vi "NI-DP_ListDevices.vi"() -> ()   [LabVIEW 2014, in "hse-network.lvlib"]
doc: "____\nHAMPEL SOFTWARE ENGINEERING v0.7.0 (2018-07-16 18:12)"
uses:
  hse-network.lvlib
panel:
  out "net address":u32
  out "name":string
  out "Devices":string[](array[string])
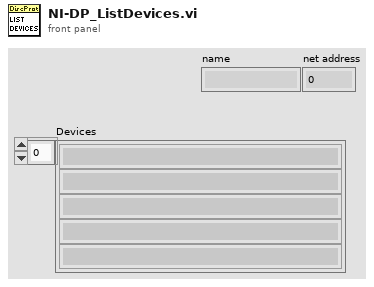
[diagram p1: front panel]
types:
  T1 = typedef "hse-network.lvlib/NI-DP__MessageStructure.ctl" = cluster{"Start of Message":string, "Command":T2, "Checksum(?) for P3,P4":string, "Always 0x02":string, "Model Code":string, "??? 1":string, "Serial":string, "Device Mac Address":string, "??? 2":string, "Param 1":string, "Param 2":string, "Param 3":string, "Param 4":string, "Checksum(?) for Network":string, "Device IP Address":string, "Device Subnet Mask":string, "Device DNS-Server":string, "Device Default Gateway":string, "??? 3":string, "End of Message":string}
  T2 = typedef "hse-network.lvlib/NI-DP__Commands.ctl" = u8
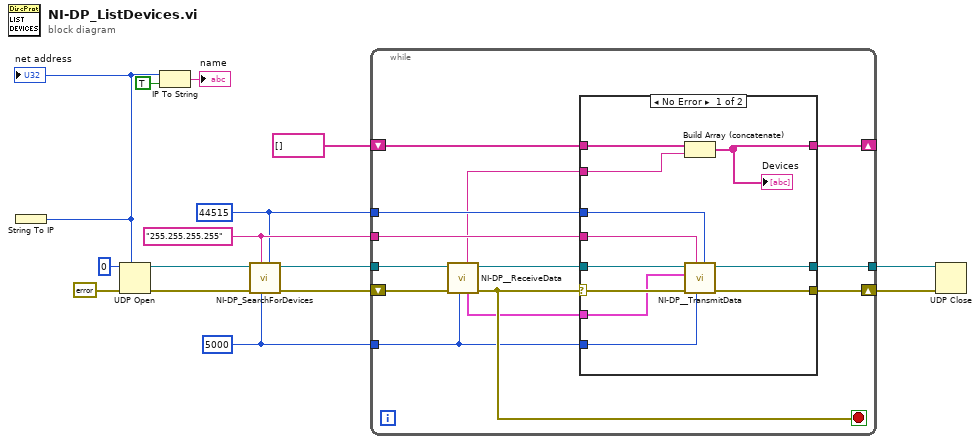
[diagram p0: block diagram]
diagram:
  w6 = u32 5000 ("timeout [ms]")
  w7 = u16 44515 ("RX Port No.")
  w8 = "255.255.255.255" ("IP to write to")
  n1 = String To IP() -> (0:w1:u32)  [unwired: 1 in]
  "net address" <- w1
  n2 = UDP Open(7:w1, 8:errorcluster {"status"=FALSE, "code"=0, "source"=""} ("error in (no error)"), 11:u16 0 ("port")) -> (port=w13:refnum<k16>, 0:w15:errorcluster)  [unwired: 2 in, 1 out]
  n3 = IP To String(1:TRUE ("dot notation? (F)"), 2:w1) -> (0:→"name":string)
  n4 = call "NI-DP_SearchForDevices.vi"("RX Port No."=w7, "timeout [ms]"=w6, "IP to write to"=w8, "error in (no error)"=w15, "UDP Network Connection in"=w13) -> ("error out"=w12:errorcluster, "UDP Network Connection out"=w11:refnum<k16>)  [unwired: 5 in]
  n5 = while {
    shift-right: [w26] -> w10
    shift-left: w12 -> [w28]
    tunnel: w11 -> [w25]
    tunnel: [w23] -> w9
    tunnel: w8 -> [w21]
    tunnel: w7 -> [w20]
    tunnel: w6 -> [w19]
    shift-right: [w18] -> _
    shift-left: string[] [] ("Array") -> [w17]
    stop <- w27 stop-if-true
    n6 = call "NI-DP__ReceiveData.vi"("timeout [ms]"=w19, "error in"=w28, "UDP Network Connection in"=w25) -> ("error out"=w27:errorcluster, "UDP Network Connection out"=w24:refnum<k16>, "UDP-NI Message"=w22:T1, "IP (MAC)"=w16:string)  [unwired: 3 in, 2 out]
    n7 = case shown="No Error" w27 {
      selector: w27 -> [w39 w41]
      tunnel: [w38 w41] -> w26
      tunnel: w24 -> [w37 w42]
      tunnel: [w36 w42] -> w23
      tunnel: w22 -> [w35 _]
      tunnel: w21 -> [w34 _]
      tunnel: w20 -> [w33 _]
      tunnel: w19 -> [w32 _]
      tunnel: [w29 w40] -> w18
      tunnel: w17 -> [w31 w40]
      tunnel: w16 -> [w30 _]
      frame No Error {
        n8 = Build Array (concatenate)(w31, w30) -> (w29:string[])
        "Devices" <- w29
        n9 = call "NI-DP__TransmitData.vi"("Port to write to"=w33, "timeout ms"=w32, "IP to write to"=w34, "error in"=w39, "UDP-NI__Message"=w35, "UDP Network Connection in"=w37) -> ("error out"=w38:errorcluster, "UDP Network Connection out"=w36:refnum<k16>)  [unwired: 4 in]
      }
      frame Error {
      }
    }
  }
  n10 = UDP Close(connection ID=w9, 8:w10) -> ()  [unwired: 2 out]
